vi "Lot End.vi"(8 "error in":errorcluster, 10 "Test Result In":T2, 11 "CalCfg File In":T1) -> (0 "error out":errorcluster, 1 "Pass":bool, 2 "Test Result Out":T2, 3 "CalCfg File Out":T1, 4 "String":string)   [LabVIEW 2020, in "GUCalibration2.lvlib"]
uses:
  GUCalibration2.lvlib
  Controls/Test Result.ctl
  Controls/Site Data Element.ctl
  Controls/Site Raw Data Element.ctl
  Controls/User Facing Msg Enum.ctl
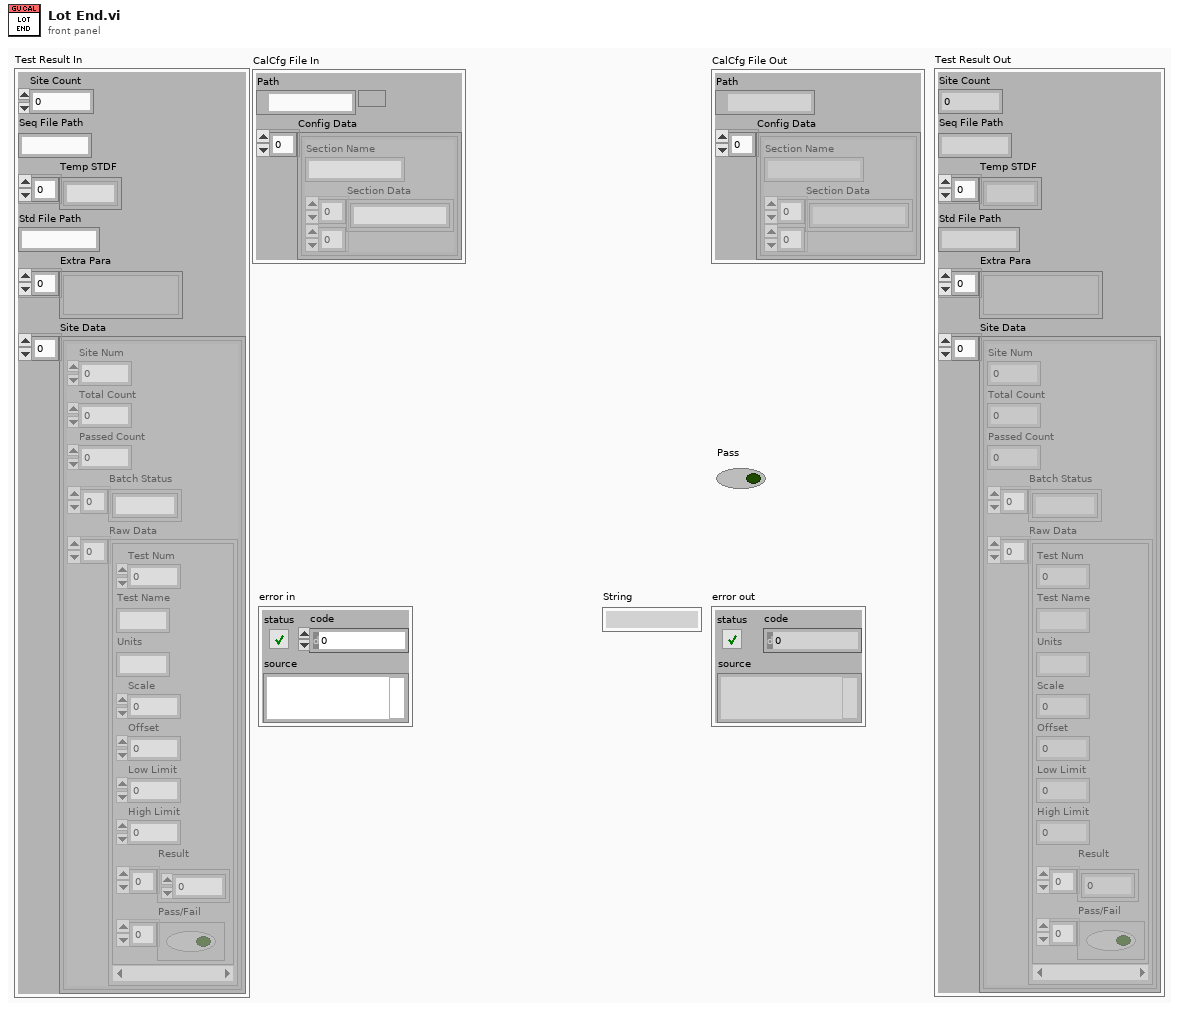
[diagram p1: front panel]
types:
  T1 = cluster{"Path":path, "Config Data":cluster{"Section Name":string, "Section Data":string[][]}[]}
  T2 = typedef "GUCalibration2.lvlib/Test Result.ctl" = cluster{"Site Count":i32, "Seq File Path":string, "Temp STDF":string[], "Std File Path":string, "Extra Para":variant[], "Site Data":T3[]}
  T3 = typedef "GUCalibration2.lvlib/Site Data Element.ctl" = cluster{"Site Num":i32, "Total Count":i32, "Passed Count":i32, "Batch Status":string[], "Raw Data":T4[]}
  T4 = typedef "GUCalibration2.lvlib/Site Raw Data Element.ctl" = cluster{"Test Num":u32, "Test Name":string, "Units":string, "Scale":i8, "Offset":dbl, "Low Limit":dbl, "High Limit":dbl, "Result":dbl[], "Pass/Fail":bool[]}
  T5 = typedef "GUCalibration2.lvlib/User Facing Msg Enum.ctl" = enum16{"Invalid GU Number", "Select More GU", "Exceptional Lot End", "Not All Sites Test", "GU Arrange Error", "Put GU In Sites", "No Cal Site Offset Msg"}
  T6 = cluster{"Section Name":string, "Section Data":string[][]}[]
  T7 = typedef "GUCalibration2.lvlib/Config Data Type.ctl" = cluster{"Cal Type":i32, "Curr Batch Index":i32, "Loop Count Per GU":i32, "Min Num of Pass GUs Per Site":i32, "Is Calibration":bool, "Batch Iteration Done":bool, "Cal Abort":bool, "Update Offset":bool, "Cal Check Pass":bool, "Cal End":bool, "Enabled Site":i32[], "GU Selected":i32[], "All Available GU":i32[], "GU Arrange":i32[][], "Batch Test Count":i32[][], "Batch Test Result":string[][], "Curr Batch":i32[], "Curr Batch Test Count":i32[], "Curr Batch Target Count":i32[], "Curr Batch Test Result":string[]}
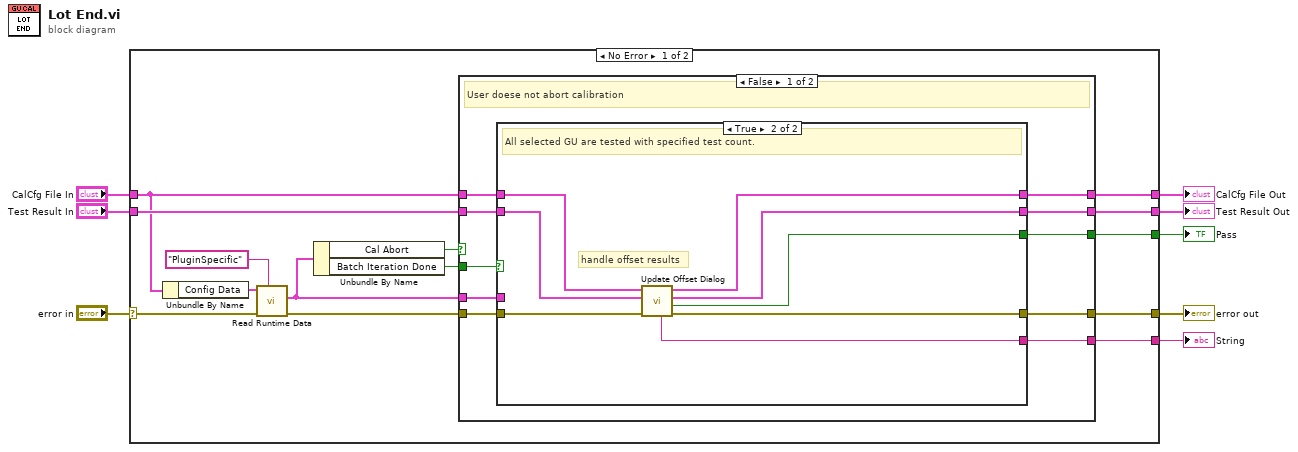
[diagram p0: block diagram]
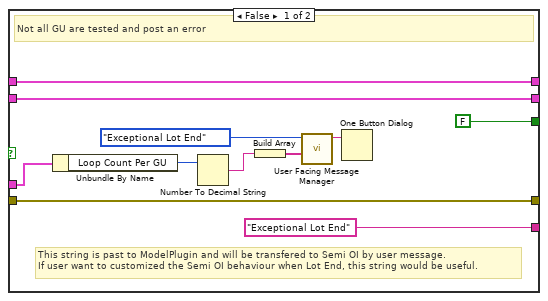
[diagram p2: hidden frame]
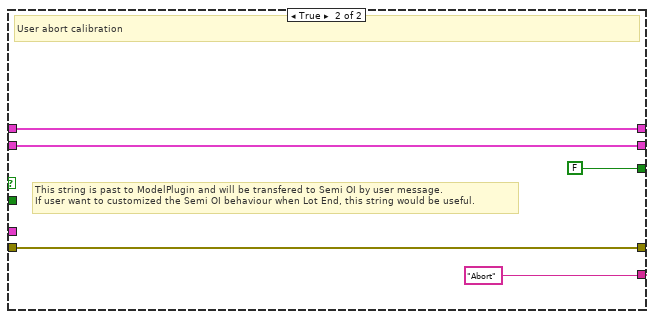
[diagram p3: hidden frame]
diagram:
  n1 = case shown="No Error" "error in" {
    selector: "error in" -> [w10 w57]
    tunnel: [w22 w57] -> w8
    tunnel: [w21 w59] -> w7
    tunnel: [w20 _] -> w6
    tunnel: [w19 w58] -> w5
    tunnel: [w18 _] -> w4
    tunnel: "Test Result In" -> [w17 w58]
    tunnel: "CalCfg File In" -> [w16 w59]
    frame No Error {
      n2 = Unbundle By Name(w16) -> ("Config Data"=w15:T6)
      n3 = call "Read Runtime Data.vi"("Section Name"="PluginSpecific", "error in"=w10, "Config File Data In"=w15) -> ("error out"=w14:errorcluster, "Runtime Data Out"=w13:T7)  [unwired: 6 in, 1 out]
      n4 = Unbundle By Name(w13) -> ("Cal Abort"=w11:bool, "Batch Iteration Done"=w12:bool)
      n5 = case shown="False" w11 {
        tunnel: [w32 w56] -> w22
        tunnel: [w31 w53] -> w21
        tunnel: [w30 FALSE ("Update OK")] -> w20
        tunnel: [w29 w52] -> w19
        tunnel: [w28 "Abort" ("Return String")] -> w18
        tunnel: w17 -> [w27 w52]
        tunnel: w16 -> [w26 w53]
        tunnel: w14 -> [w25 w56]
        tunnel: w13 -> [w24 _]
        tunnel: w12 -> [w23 _]
        frame False {
          # "User doese not abort calibration"
          n6 = case shown="True" w23 {
            tunnel: [w33 w45] -> w32
            tunnel: [w42 w48] -> w31
            tunnel: [FALSE ("Update OK") w46] -> w30
            tunnel: [w43 w47] -> w29
            tunnel: ["Exceptional Lot End" ("Return String") w44] -> w28
            tunnel: w27 -> [w43 w49]
            tunnel: w26 -> [w42 w50]
            tunnel: w25 -> [w33 w51]
            tunnel: w24 -> [w41 _]
            frame False {
              # "This string is past to ModelPlugin and will be transfered to Semi OI by user message.\nIf user want to customized the Semi OI behaviour when Lot End, this string would be useful."
              # "Not all GU are tested and post an error"
              n7 = Unbundle By Name(w41) -> ("Loop Count Per GU"=w36:i32)
              n8 = Number To Decimal String(number=w36) -> (decimal integer string=w35:string)  [unwired: 1 in]
              n9 = Build Array(w35) -> (w34:string[])
              n10 = call "User Facing Message Manager.vi"("Variable Msg"=w34, "User Facing Msg"=User_Facing_Msg_Enum."Exceptional Lot End") -> ("User Facing Msg Out"=w37:string)  [unwired: 7 in, 2 out]
              n11 = One Button Dialog(message=w37) -> ()  [unwired: 1 in, 1 out]
            }
            frame True {
              # "handle offset results"
              # "All selected GU are tested with specified test count."
              n12 = call "Update Offset Dialog.vi"("error in"=w51, "Test Result In"=w49, "CalCfg File In"=w50) -> ("error out"=w45:errorcluster, "Pass"=w46:bool, "Test Result Out"=w47:T2, "CalCfg File Out"=w48:T1, "String"=w44:string)  [unwired: 4 in]
            }
          }
        }
        frame True {
          # "This string is past to ModelPlugin and will be transfered to Semi OI by user message.\nIf user want to customized the Semi OI behaviour when Lot End, this string would be useful."
          # "User abort calibration"
        }
      }
    }
    frame Error {
    }
  }
  "error out" <- w8
  "Pass" <- w6
  "Test Result Out" <- w5
  "CalCfg File Out" <- w7
  "String" <- w4
